vi "1D_to_2D.vi"() -> ()   [LabVIEW 2017]
panel:
  out "Array 2":u32[](array[colorbox])=[15463629, 16769393, 2837841, 16753544, 10003068]
  out "size(s)":i32
  out "Array":u32[][](array[colorbox])=[[15463629, 16769393, 2837841, 16753544, 10003068]]
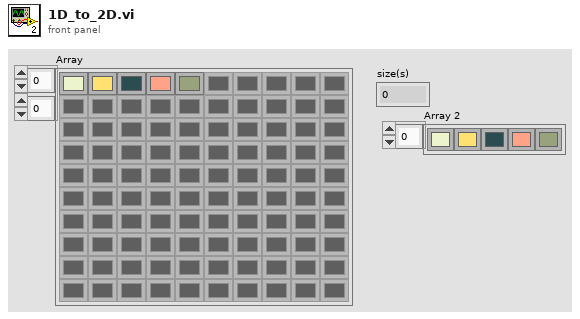
[diagram p1: front panel]
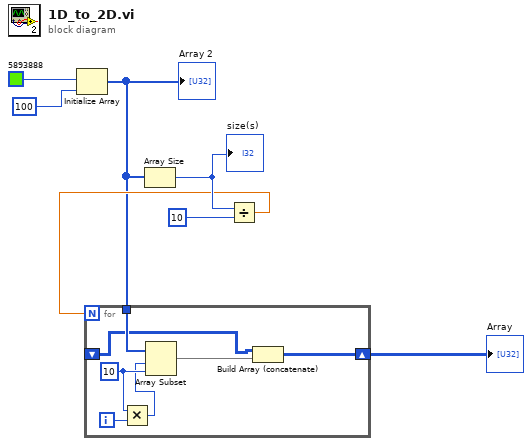
[diagram p0: block diagram]
diagram:
  n1 = Initialize Array "Initialize Array"(u32 5893888, 100 ("dimension size")) -> (w2:u32[])
  "Array 2" <- w2
  n2 = Array Size(array=w2) -> (size(s)=w7:i32)
  "size(s)" <- w7
  n3 = Divide(x=w7, y=10) -> (x/y=w5:dbl)
  n4 = for {
    N: w5 -> [_]
    tunnel: w2 -> [w11]
    shift-right: [w10] -> w1
    shift-left: _ -> [w8]
    i -> [w14]
    w13 = 10 ("length")
    n5 = Multiply(x=w13, y=w14) -> (x*y=w12:i32)
    n6 = Array Subset "Array Subset"(array=w11, index=w12, length=w13) -> (w9:u32[])
    n7 = Build Array (concatenate)(w8, w9) -> (w10:u32[][])
  }
  "Array" <- w1
